vi "Get Request Events.vi"(8 "error in":errorcluster, 11 "Create new?":bool) -> (0 "error out":errorcluster, 3 "Request Events":T1)   [LabVIEW 2014, in "Chart Module.lvlib"]
uses:
  Chart Module.lvlib
  Request Events--cluster.ctl
  Stop Argument--cluster.ctl
  Show Panel Argument--cluster.ctl
  Hide Panel Argument--cluster.ctl
  Limits Argument--cluster.ctl
  Send Value Argument--cluster.ctl
  Clear Chart--arguments.ctl
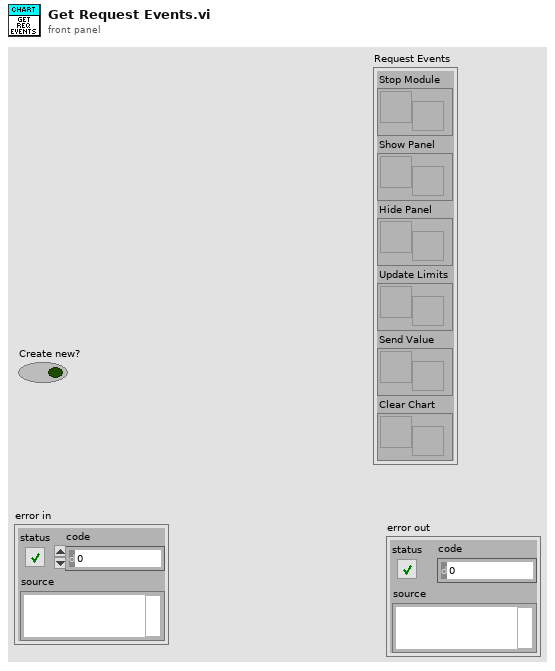
[diagram p1: front panel]
types:
  T1 = typedef "Chart Module.lvlib/Request Events--cluster.ctl" = cluster{"Stop Module":refnum<user-event>, "Show Panel":refnum<user-event>, "Hide Panel":refnum<user-event>, "Update Limits":refnum<user-event>, "Send Value":refnum<user-event>, "Clear Chart":refnum<user-event>}
  T2 = typedef "Chart Module.lvlib/Clear Chart--arguments.ctl" = cluster{"Clear Chart?":bool}
  T3 = typedef "Chart Module.lvlib/Send Value Argument--cluster.ctl" = cluster{"Value":dbl}
  T4 = typedef "Chart Module.lvlib/Limits Argument--cluster.ctl" = cluster{"Enabled?":bool, "HighLim":dbl, "LowLim":dbl}
  T5 = typedef "Chart Module.lvlib/Hide Panel Argument--cluster.ctl" = cluster{"Hide Panel?":bool}
  T6 = typedef "Chart Module.lvlib/Show Panel Argument--cluster.ctl" = cluster{"Show Panel?":bool}
  T7 = typedef "Chart Module.lvlib/Stop Argument--cluster.ctl" = cluster{"Origin":string, "Exit via Stop Module Req?":bool}
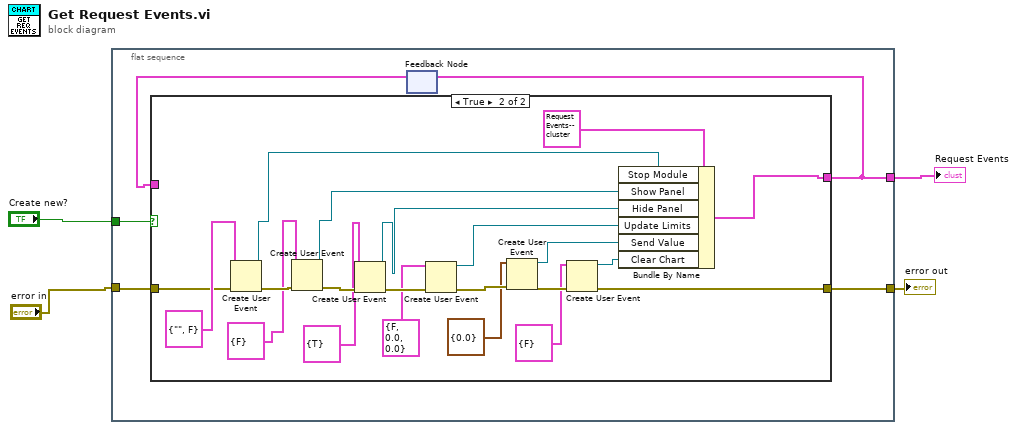
[diagram p0: block diagram]
diagram:
  n1 = flat-sequence {
    tunnel: "Create new?" -> [w9]
    tunnel: [w8] -> w3
    tunnel: "error in" -> [w7]
    tunnel: [w6] -> w1
    frame #0 {
      n2 = feedback #1() -> (w5:T1)  [unwired: 1 in]
      n3 = case shown="True" w9 {
        tunnel: [w10 w14] -> w8
        tunnel: w7 -> [w10 w30]
        tunnel: [w11 w16] -> w6
        tunnel: w5 -> [w11 _]
        frame False {
        }
        frame True {
          n4 = Create User Event(user event datatype=T7 {"Origin"="", "Exit via Stop Module Req?"=FALSE} ("Stop Argument"), error in=w30) -> (user event=w28:refnum<user-event>, error out=w31:errorcluster)
          n5 = Create User Event(user event datatype=T6 {"Show Panel?"=FALSE} ("Show Panel Argument"), error in=w31) -> (user event=w19:refnum<user-event>, error out=w27:errorcluster)
          n6 = Create User Event(user event datatype=T5 {"Hide Panel?"=TRUE} ("Hide Panel Argument"), error in=w27) -> (user event=w23:refnum<user-event>, error out=w25:errorcluster)
          n7 = Create User Event(user event datatype=T4 {"Enabled?"=FALSE, "HighLim"=0.0, "LowLim"=0.0} ("Limits Argument"), error in=w25) -> (user event=w20:refnum<user-event>, error out=w22:errorcluster)
          n8 = Create User Event(user event datatype=T3 {"Value"=0.0} ("Send Value Argument"), error in=w22) -> (user event=w15:refnum<user-event>, error out=w18:errorcluster)
          n9 = Create User Event(user event datatype=T2 {"Clear Chart?"=FALSE} ("Clear Chart Arguments"), error in=w18) -> (user event=w12:refnum<user-event>, error out=w14:errorcluster)
          n10 = Bundle By Name(cluster=T1 {"Stop Module"=refnum, "Show Panel"=refnum, "Hide Panel"=refnum, "Update Limits"=refnum, "Send Value"=refnum, "Clear Chart"=refnum} ("Request Events"), "Stop Module"=w28, "Show Panel"=w19, "Hide Panel"=w23, "Update Limits"=w20, "Send Value"=w15, "Clear Chart"=w12) -> (w16:T1)
        }
      }
      n11 = feedback-in #1(w6) -> ()
    }
  }
  "error out" <- w3
  "Request Events" <- w1
